vi "initial.vi"(8 "error in (no error)":errorcluster, 10 "Path":path, 11 "TXT in":refnum<class "TXT.lvclass">) -> (0 "error out":errorcluster, 3 "TXT out":refnum<class "TXT.lvclass">)   [LabVIEW 2014, in "TXT.lvclass"]
uses:
  TXT.lvclass
  TXT.lvclass/TXT.ctl
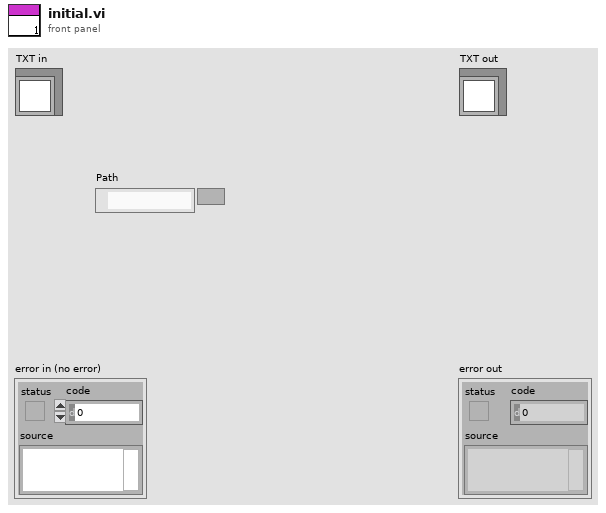
[diagram p1: front panel]
types:
  T1 = enum16{"open", "replace", "create", "open or create", "replace or create", "replace or create with confirmation"}
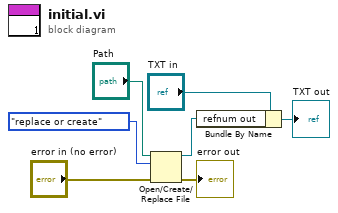
[diagram p0: block diagram]
diagram:
  n1 = Open/Create/Replace File(file path (use dialog)="Path", error in="error in (no error)", operation (0:open)=T1."replace or create") -> (refnum out=w2:refnum<file>, error out=→"error out":errorcluster)  [unwired: 3 in, 1 out]
  n2 = Bundle By Name(cluster="TXT in", "refnum out"=w2) -> (→"TXT out":refnum<class "TXT.lvclass">)
